vi "new.vi"(4 "output range":cluster{"output high":dbl, "output low":dbl}={"output high"=100.0, "output low"=-100.0} {"output low" format="%.2f"; "output high" format="%.2f"}, 5 "setpoint":dbl format="%.2f", 6 "dt (s)":dbl=-1.0 format="%.3f", 7 "process variable":dbl format="%.2f", 9 "Initial integrated error":dbl, 10 "reinitialize? (F)":bool, 11 "PID gains":T1={"proportional gain (Kc)"=1.0, "integral time (Ti, min)"=0.01, "derivative time (Td, min)"=0.0} {"derivative time (Td, min)" format="%.3f"; "integral time (Ti, min)" format="%.3f"; "proportional gain (Kc)" format="%.3f"}) -> (2 "dt out (s)":dbl format="%.3f", 3 "output":dbl format="%.2f")   [LabVIEW 2016]
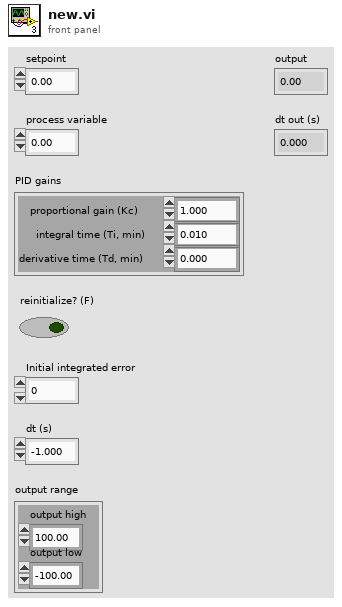
[diagram p1: front panel]
types:
  T1 = cluster{"proportional gain (Kc)":dbl, "integral time (Ti, min)":dbl, "derivative time (Td, min)":dbl}
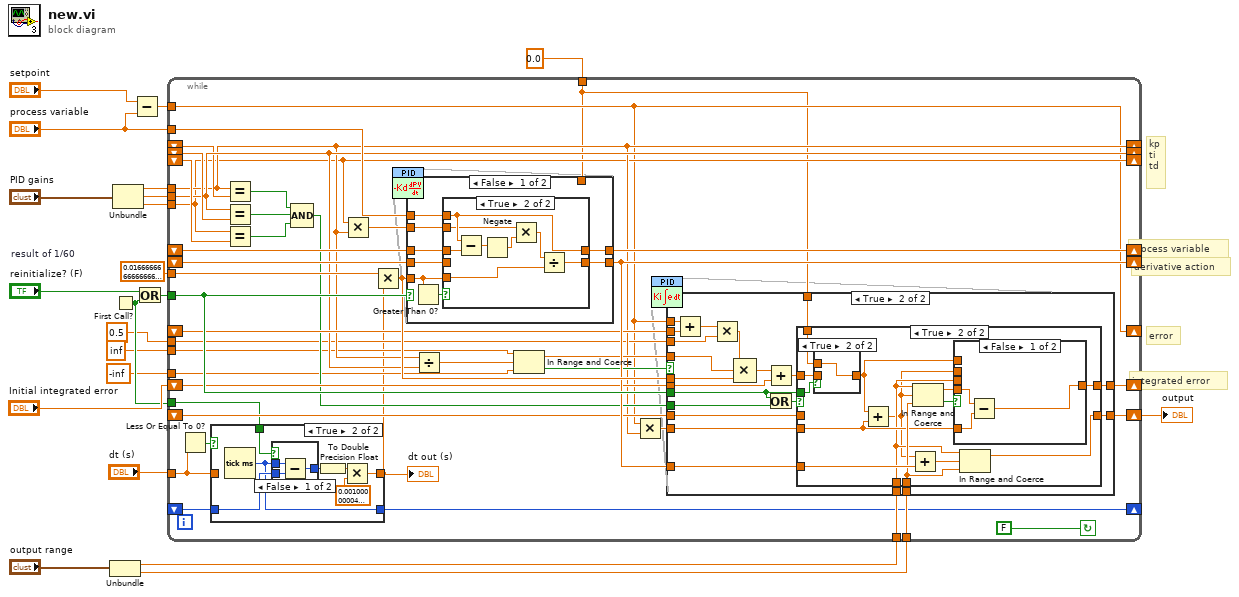
[diagram p0: block diagram]
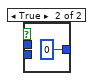
[diagram p3: hidden frame]
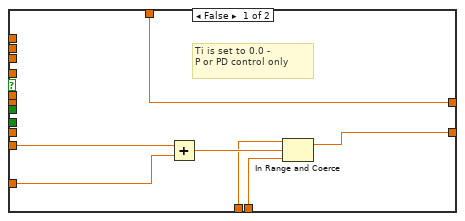
[diagram p4: hidden frame]
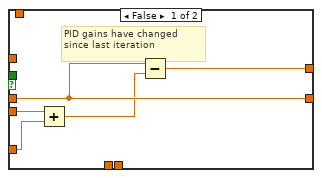
[diagram p5: hidden frame]
diagram:
  w7 = 0.016666666666666666  # result of 1/60
  # "derivative action"
  # "process variable"
  # "kp\nti\ntd"
  # "error"
  # "integrated error"
  n1 = Unbundle("output range") -> ("output high"=w5:dbl, "output low"=w6:dbl)
  n2 = First Call?() -> (First Call?: T/F=w20:bool)
  n3 = Unbundle("PID gains") -> ("proportional gain (Kc)"=w2:dbl, "integral time (Ti, min)"=w3:dbl, "derivative time (Td, min)"=w4:dbl)
  n4 = Subtract(x="setpoint", y="process variable") -> (x-y=w18:dbl)
  n5 = Or(x="reinitialize? (F)", y=w20) -> (x .or. y?=w1:bool)
  n6 = while {
    tunnel: w1 -> [w63]
    shift-left: _ -> [w25]
    shift-right: [w26] -> _
    shift-right: [w35] -> _
    shift-left: _ -> [w36]
    shift-right: [w37] -> _
    shift-left: _ -> [w60]
    shift-right: [w30] -> _
    shift-left: _ -> [w61]
    tunnel: w2 -> [w35]
    tunnel: w3 -> [w37]
    tunnel: w4 -> [w30]
    tunnel: "dt (s)" -> [w24]
    tunnel: w5 -> [w56]
    tunnel: w6 -> [w55]
    tunnel: "process variable" -> [w54]
    shift-right: [w53] -> _
    shift-left: _ -> [w52]
    shift-right: [w51] -> _
    shift-left: _ -> [w43]
    shift-right: [w50] -> w14
    shift-left: _ -> [w49]
    shift-right: [w29] -> _
    shift-left: _ -> [w48]
    shift-right: [w47] -> _
    shift-left: "Initial integrated error" -> [w46]
    tunnel: w7 -> [w40]
    tunnel: 0.5 ("y") -> [w34]
    tunnel: inf ("upper limit") -> [w32]
    tunnel: -inf ("lower limit") -> [w33]
    tunnel: w18 -> [w29]
    tunnel: 0.0 -> [w28]
    tunnel: w20 -> [w22]
    stop <- FALSE continue-if-true
    n7 = Less Or Equal To 0?(x=w24) -> (x <= 0?=w23:bool)
    n8 = case shown="True" w23 {
      tunnel: [w65 w69] -> w27
      tunnel: w25 -> [w64 w68]
      tunnel: [w64 w67] -> w26
      tunnel: w24 -> [w65 _]
      tunnel: w22 -> [_ w66]
      frame False {
      }
      frame True {
        n9 = Tick Count (ms)() -> (millisecond timer value=w67:u32)
        n10 = case shown="False" w66 {
          tunnel: [w75 u32 0] -> w71
          tunnel: w68 -> [w74 _]
          tunnel: w67 -> [w73 _]
          frame False {
            n11 = Subtract(x=w73, y=w74) -> (x-y=w75:u32)
          }
          frame True {
          }
        }
        n12 = To Double Precision Float(number=w71) -> (double precision float=w70:dbl)
        n13 = Multiply(x=w70, y=0.0010000000474974513) -> (x*y=w69:dbl)
      }
    }
    "dt out (s)" <- w27
    n14 = Equal?(x=w35, y=w36) -> (x = y?=w58:bool)
    n15 = Equal?(x=w37, y=w60) -> (x = y?=w57:bool)
    n16 = Equal?(x=w30, y=w61) -> (x = y?=w59:bool)
    n17 = Compound Arithmetic op=AND(w58, w57, w59) -> (w38:bool)
    n18 = Multiply(x=w30, y=w35) -> (x*y=w42:dbl)
    n19 = Multiply(x=w40, y=w27) -> (x*y=w62:dbl)
    n20 = case shown="False" w63 {
      tunnel: w52 -> [w137 _]
      tunnel: w42 -> [w134 _]
      tunnel: w54 -> [w136 w149]
      tunnel: [w133 w149] -> w53
      tunnel: [w135 w148] -> w51
      tunnel: w43 -> [w131 _]
      tunnel: w62 -> [w130 _]
      tunnel: w28 -> [_ w148]
      frame False {
        n21 = Greater Than 0?(x=w130) -> (x > 0?=w132:bool)
        n22 = case shown="True" w132 {
          tunnel: w137 -> [w139 w145]
          tunnel: w130 -> [_ w144]
          tunnel: w136 -> [_ w142]
          tunnel: [w138 w143] -> w135
          tunnel: w134 -> [_ w140]
          tunnel: [w139 w142] -> w133
          tunnel: w131 -> [w138 _]
          frame False {
            # "dt = 0 min"
          }
          frame True {
            n23 = Subtract(x=w142, y=w145) -> (x-y=w147:dbl)
            n24 = Negate(x=w147) -> (-x=w141:dbl)
            n25 = Multiply(x=w140, y=w141) -> (x*y=w146:dbl)
            n26 = Divide(x=w146, y=w144) -> (x/y=w143:dbl)
          }
        }
      }
      frame True {
      }
    }
    n27 = Divide(x=w35, y=w37) -> (x/y=w41:dbl)
    n28 = In Range and Coerce(upper limit=w32, x=w41, lower limit=w33) -> (coerced(x)=w45:dbl, In Range?=w44:bool)
    n29 = Multiply(x=w29, y=w35) -> (x*y=w39:dbl)
    n30 = case shown="True" w44 {
      tunnel: w29 -> [_ w103]
      tunnel: w48 -> [_ w104]
      tunnel: w46 -> [_ w99]
      tunnel: [w77 w94] -> w47
      tunnel: w45 -> [_ w92]
      tunnel: w39 -> [w82 w97]
      tunnel: [w83 w93] -> w50
      tunnel: w49 -> [_ w95]
      tunnel: w51 -> [w81 w91]
      tunnel: w63 -> [_ w90]
      tunnel: w38 -> [_ w89]
      tunnel: w62 -> [_ w88]
      tunnel: w56 -> [w79 w86]
      tunnel: w55 -> [w78 w87]
      tunnel: w34 -> [_ w85]
      tunnel: w28 -> [w77 w84]
      frame False {
        # "Ti is set to 0.0 -\nP or PD control only"
        n31 = Add(x=w82, y=w81) -> (x+y=w80:dbl)
        n32 = In Range and Coerce(upper limit=w79, x=w80, lower limit=w78) -> (coerced(x)=w83:dbl)  [unwired: 1 out]
      }
      frame True {
        n33 = Add(x=w103, y=w104) -> (x+y=w102:dbl)
        n34 = Multiply(x=w102, y=w85) -> (x*y=w101:dbl)
        n35 = Compound Arithmetic op=MULTIPLY(w101, w92, w88) -> (w100:dbl)
        n36 = Add(x=w100, y=w99) -> (x+y=w98:dbl)
        n37 = Or(x=w90, y=w89) -> (x .or. y?=w96:bool)
        n38 = case shown="True" w96 {
          tunnel: w98 -> [_ w117]
          tunnel: w97 -> [w107 w112]
          tunnel: w95 -> [w109 _]
          tunnel: w90 -> [_ w119]
          tunnel: [w108 w114] -> w94
          tunnel: [w109 w122] -> w93
          tunnel: w91 -> [w106 w121]
          tunnel: w87 -> [_ w120]
          tunnel: w86 -> [_ w111]
          tunnel: w84 -> [_ w118]
          frame False {
            # "PID gains have changed\nsince last iteration"
            n39 = Add(x=w107, y=w106) -> (x+y=w105:dbl)
            n40 = Subtract(x=w109, y=w105) -> (x-y=w108:dbl)
          }
          frame True {
            n41 = case shown="True" w119 {
              tunnel: w118 -> [_ w129]
              tunnel: [w128 w129] -> w116
              tunnel: w117 -> [w128 _]
              frame False {
              }
              frame True {
              }
            }
            n42 = Add(x=w116, y=w112) -> (x+y=w110:dbl)
            n43 = Add(x=w110, y=w121) -> (x+y=w123:dbl)
            n44 = In Range and Coerce(upper limit=w111, x=w110, lower limit=w120) -> (coerced(x)=w113:dbl, In Range?=w115:bool)
            n45 = case shown="False" w115 {
              tunnel: w116 -> [_ w127]
              tunnel: [w124 w127] -> w114
              tunnel: w113 -> [w126 _]
              tunnel: w112 -> [w125 _]
              tunnel: w111 -> [_ _]
              tunnel: w110 -> [_ _]
              frame False {
                n46 = Subtract(x=w126, y=w125) -> (x-y=w124:dbl)
              }
              frame True {
              }
            }
            n47 = In Range and Coerce(upper limit=w111, x=w123, lower limit=w120) -> (coerced(x)=w122:dbl)  [unwired: 1 out]
          }
        }
      }
    }
  }
  "output" <- w14
